vi "Configure Timebase.vi"(6 "Maximum Sample Points (500)":i32(ring)=500 items=["50"=50, "100"=100, "250"=250, "500"=500, "1000"=1000, "2500"=2500, "5K"=5000, "10K"=10000, "25K"=25000, "50K"=50000, "100K"=100000, "250K"=250000, "500K"=500000, "1M"=1000000, "2M"=2000000, "2.5M"=2500000, "5M"=5000000, "10M"=10000000, "25M"=25000000, "50M"=50000000, "100M"=100000000], 8 "error in (no error)":errorcluster, 9 "Position (0.0 s)":dbl, 10 "Timebase (0.0005 s)":dbl=0.0005, 11 "VISA resource name":refnum<visa-resource-name>) -> (0 "error out":errorcluster, 3 "VISA resource name out":refnum<visa-resource-name>)   [LabVIEW 2015, in "LeCroy Wave Series.lvlib"]
doc: "Configures the timebase and horizontal features of the oscilloscope."
uses:
  <instrlib>/LeCroy Wave Series/LeCroy Wave Series.lvlib
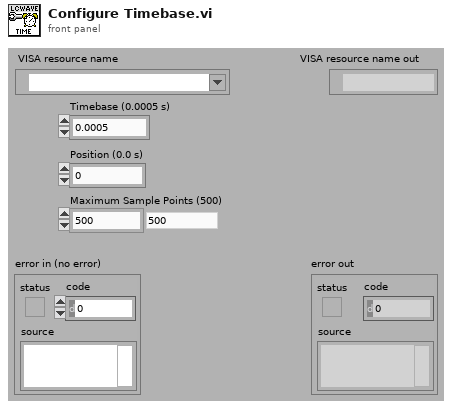
[diagram p1: front panel]
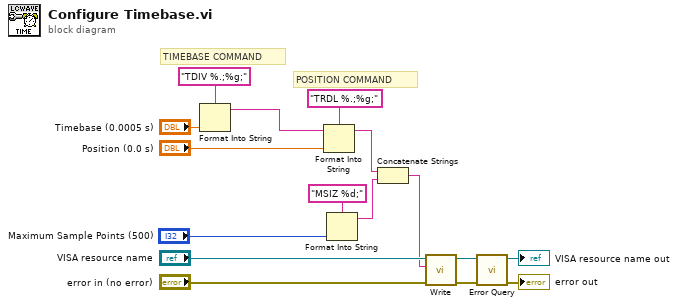
[diagram p0: block diagram]
diagram:
  # "POSITION COMMAND"
  # "TIMEBASE COMMAND"
  n1 = Format Into String(format string="TDIV %.;%g;", "Timebase (0.0005 s)") -> (resulting string=w11:string)  [unwired: 2 in, 1 out]
  n2 = Format Into String(format string="TRDL %.;%g;", initial string=w11, "Position (0.0 s)") -> (resulting string=w5:string)  [unwired: 1 in, 1 out]
  n3 = Format Into String(format string="MSIZ %d;", "Maximum Sample Points (500)") -> (resulting string=w1:string)  [unwired: 2 in, 1 out]
  n4 = Concatenate Strings(w5, w1) -> (w4:string)
  n5 = call <instrlib>:"Write.vi"("error in (no error)"="error in (no error)", "Write Buffer"=w4, "VISA resource name"="VISA resource name") -> ("error out"=w8:errorcluster, "VISA resource name out"=w9:refnum<visa-resource-name>)  [unwired: 6 in, 1 out]
  n6 = call <instrlib>:"Error Query.vi"("error in (no error)"=w8, "VISA resource name"=w9) -> ("error out"=→"error out":errorcluster, "VISA resource name out"=→"VISA resource name out":refnum<visa-resource-name>)  [unwired: 6 in, 2 out]
